vi "加标回收数据处理整合 (子VI).vi"(11 "枚举":enum16{"实时数据排序", "小时数据排序"}(ring)) -> (3 "已排序的数组":string[](array[string]))   [LabVIEW 2016, in "数据传输系统-04.lvlib"]
uses:
  <userlib>/_OpenG.lib/array/array.llb/Remove Duplicates from 1D Array (String)__ogtk.vi
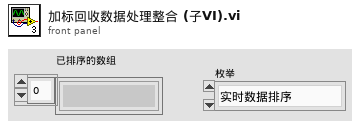
[diagram p1: front panel]
types:
  T1 = cluster{"PH":string[][], "CODCr":string[][], "氨氮":string[][], "CODMn":string[][], "总氮":string[][], "总磷":string[][], "电导率":string[][], "水温":string[][], "COD":string[][], "DO":string[][], "浊度":string[][], "叶绿素":string[][], "藻密度":string[][], "铜":string[][], "盐度":string[][], "水位":string[][], "流速":string[][], "方向":string[][], "瞬时流量":string[][], "累积流量":string[][], "正累积流量":string[][], "负累积流量":string[][], "亚硝酸盐":string[][], "硫化物":string[][], "ORP":string[][], "铅":string[][], "镉":string[][], "锌":string[][], "镍":string[][], "锰":string[][], "汞":string[][], "气温":string[][], "气压":string[][], "风速":string[][], "风向":string[][], "空气温度":string[][], "相对湿度":string[][], "分钟雨量":string[][], "小时雨量":string[][], "日雨量":string[][], "累积雨量":string[][], "盐度":string[][], "磷酸盐":string[][], "硝氮":string[][], "氟化物":string[][], "挥发酚":string[][], "氯化物":string[][], "蓝绿藻":string[][], "余氯":string[][], "综合生物毒性":string[][], "水深":string[][]}
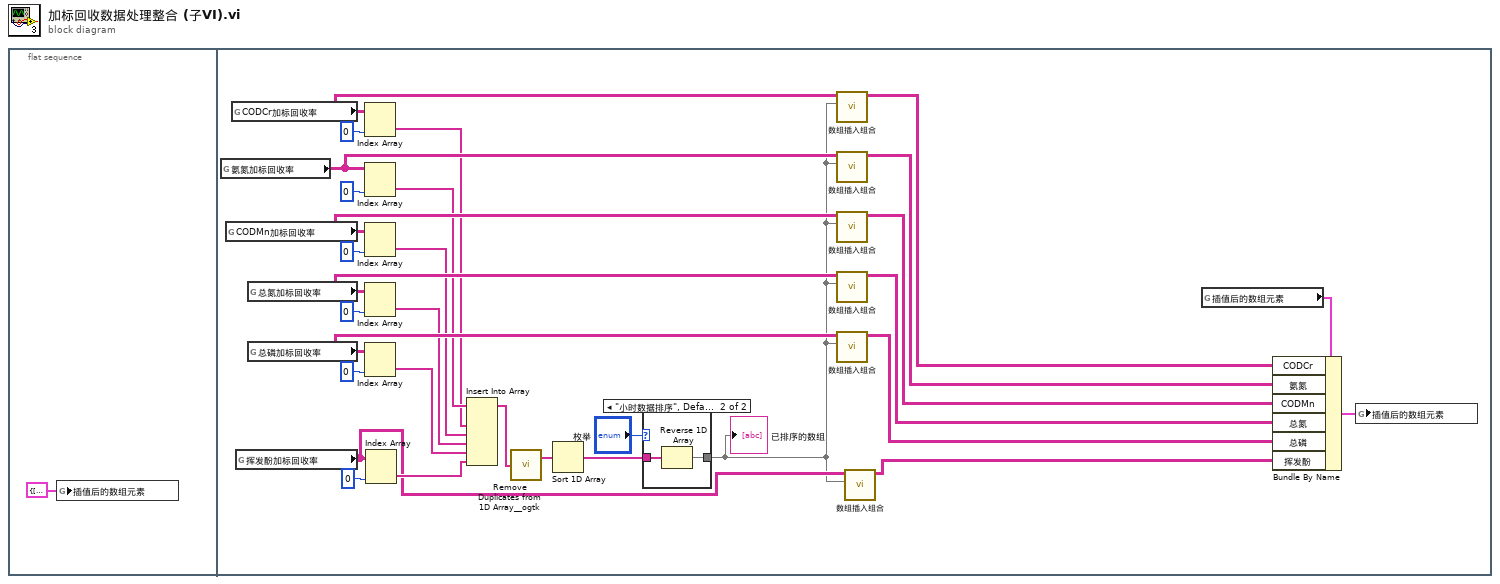
[diagram p0: block diagram]
diagram:
  n1 = flat-sequence {
    frame #0 {
      n2 = global write "插值后的新数组.vi" "插值后的数组元素"(T1 {"PH"=[], "CODCr"=[], "氨氮"=[], "CODMn"=[], "总氮"=[], "总磷"=[], "电导率"=[], "水温"=[], "COD"=[], "DO"=[], "浊度"=[], "叶绿素"=[], "藻密度"=[], "铜"=[], "盐度"=[], "水位"=[], "流速"=[], "方向"=[], "瞬时流量"=[], "累积流量"=[], "正累积流量"=[], "负累积流量"=[], "亚硝酸盐"=[], "硫化物"=[], "ORP"=[], "铅"=[], "镉"=[], "锌"=[], "镍"=[], "锰"=[], "汞"=[], "气温"=[], "气压"=[], "风速"=[], "风向"=[], "空气温度"=[], "相对湿度"=[], "分钟雨量"=[], "小时雨量"=[], "日雨量"=[], "累积雨量"=[], "盐度"=[], "磷酸盐"=[], "硝氮"=[], "氟化物"=[], "挥发酚"=[], "氯化物"=[], "蓝绿藻"=[], "余氯"=[], "综合生物毒性"=[], "水深"=[]} ("插值后的数组元素")) -> ()
    }
    frame #1 {
      n3 = global read "全局 所有参数.vi" "氨氮加标回收率"() -> (w14:string[][])
      n4 = global read "全局 所有参数.vi" "CODMn加标回收率"() -> (w25:string[][])
      n5 = global read "全局 所有参数.vi" "CODCr加标回收率"() -> (w24:string[][])
      n6 = global read "全局 所有参数.vi" "挥发酚加标回收率"() -> (w4:string[][])
      n7 = global read "全局 所有参数.vi" "总氮加标回收率"() -> (w26:string[][])
      n8 = global read "全局 所有参数.vi" "总磷加标回收率"() -> (w27:string[][])
      n9 = Index Array(array=w24, index (col)=0 ("索引 (行)")) -> (element=w12:string[])  [unwired: 1 in]
      n10 = Index Array(array=w14, index (col)=0 ("索引 (行)")) -> (element=w13:string[])  [unwired: 1 in]
      n11 = Index Array(array=w25, index (col)=0 ("索引 (行)")) -> (element=w11:string[])  [unwired: 1 in]
      n12 = Index Array(array=w26, index (col)=0 ("索引 (行)")) -> (element=w10:string[])  [unwired: 1 in]
      n13 = Index Array(array=w27, index (col)=0 ("索引 (行)")) -> (element=w9:string[])  [unwired: 1 in]
      n14 = Index Array(array=w4, index (col)=0 ("索引 (行)")) -> (element=w5:string[])  [unwired: 1 in]
      n15 = Insert Into Array(array=w13, new element #1=w12, new element #2=w11, new element #3=w10, new element #4=w9, new element #5=w5) -> (w23:string[])  [unwired: 1 in]
      n16 = call-poly <userlib>:"Remove Duplicates from 1D Array__ogtk.vi"("Input Array"=w23) -> ("Output Array"=w22:string[])  [unwired: 1 out]
      n17 = Sort 1D Array(array=w22) -> (sorted array=w15:string[])
      n18 = case shown="\"小时数据排序\", Default" "枚举" {
        tunnel: w15 -> [w33 w35]
        tunnel: [w33 w34] -> w3
        frame "实时数据排序" {
        }
        frame "小时数据排序", Default {
          n19 = Reverse 1D Array(array=w35) -> (reversed array=w34:string[])
        }
      }
      "已排序的数组" <- w3
      n20 = call "数组插入组合.vi"("排序后的一维数组"=w3, "输入数组"=w24) -> ("输出结果"=w28:string[][])  [unwired: 9 in]
      n21 = call "数组插入组合.vi"("排序后的一维数组"=w3, "输入数组"=w14) -> ("输出结果"=w29:string[][])  [unwired: 9 in]
      n22 = call "数组插入组合.vi"("排序后的一维数组"=w3, "输入数组"=w25) -> ("输出结果"=w30:string[][])  [unwired: 9 in]
      n23 = call "数组插入组合.vi"("排序后的一维数组"=w3, "输入数组"=w26) -> ("输出结果"=w31:string[][])  [unwired: 9 in]
      n24 = call "数组插入组合.vi"("排序后的一维数组"=w3, "输入数组"=w27) -> ("输出结果"=w32:string[][])  [unwired: 9 in]
      n25 = call "数组插入组合.vi"("排序后的一维数组"=w3, "输入数组"=w4) -> ("输出结果"=w2:string[][])  [unwired: 9 in]
      n26 = global read "插值后的新数组.vi" "插值后的数组元素"() -> (w8:T1)
      n27 = Bundle By Name(cluster=w8, "CODCr"=w28, "氨氮"=w29, "CODMn"=w30, "总氮"=w31, "总磷"=w32, "挥发酚"=w2) -> (w7:T1)
      n28 = global write "插值后的新数组.vi" "插值后的数组元素"(w7) -> ()
    }
  }
